vi "Start Kernel and Connect.vi"(6 "run minimized? (F)":bool=TRUE, 8 "error in (no error)":errorcluster, 9 "args":string="kernel   -f ", 10 "Path to Kernel Command (IPython)":string="\n", 11 "object in":refnum<class "JuPyter_Client.lvclass">) -> (0 "error out":errorcluster, 3 "object out":refnum<class "JuPyter_Client.lvclass">)   [LabVIEW 2018, in "JuPyter_Client.lvclass"]
doc: "Connect to an existing kernel"
uses:
  JuPyter_Client.lvclass
  Utility/Connection.ctl
  JuPyter_Client.lvclass/JuPyter_Client.ctl
  <vilib>/addons/zeromq/socket_type.ctl
  <vilib>/addons/zeromq/socket_options.ctl
  <vilib>/addons/zeromq/zmq_socket.lvclass
  <vilib>/addons/zeromq/zmq_context.lvclass
  <vilib>/addons/zeromq/zeromq.lvlib
  ClientMessaging.lvlib
  <vilib>/JDP Science/JSONtext/JSONtext.lvlib
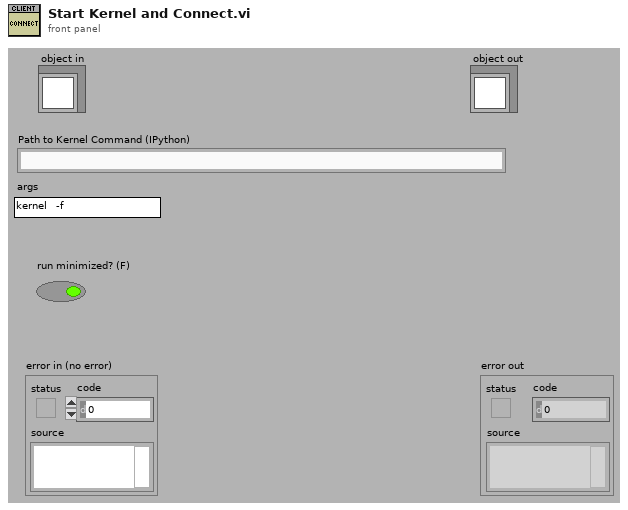
[diagram p1: front panel]
types:
  T1 = typedef "ClientMessaging.lvlib/Connection.ctl" = cluster{"transport":string, "ip":string, "key":string, "signature_scheme":string, "kernel_name":string, "shell_port":u16, "iopub_port":u16, "stdin_port":u16, "control_port":u16, "hb_port":u16}
  T2 = enum16{"Shell", "IOPub", "Stdin", "Control", "Heart Beat"}
  T3 = typedef "zeromq.lvlib/socket_type.ctl" = enum8{"ZMQ_PAIR", "ZMQ_PUB", "ZMQ_SUB", "ZMQ_REQ", "ZMQ_REP", "ZMQ_DEALER", "ZMQ_ROUTER", "ZMQ_PULL", "ZMQ_PUSH", "ZMQ_XPUB", "ZMQ_XSUB"}
  T4 = typedef "zeromq.lvlib/socket_options.ctl" = enum8{"NONE", "ZMQ_HWM", "<2>", "ZMQ_SWAP", "ZMQ_AFFINITY", "ZMQ_IDENTITY", "ZMQ_SUBSCRIBE", "ZMQ_UNSUBSCRIBE", "ZMQ_RATE", "ZMQ_RECOVERY_IVL", "ZMQ_MCAST_LOOP", "ZMQ_SNDBUF", "ZMQ_RCVBUF", "ZMQ_RCVMORE", "ZMQ_FD", "ZMQ_EVENTS", "ZMQ_TYPE", "ZMQ_LINGER", "ZMQ_RECONNECT_IVL", "ZMQ_BACKLOG", "ZMQ_RECOVERY_IVL_MSEC", "ZMQ_RECONNECT_IVL_MAX", "ZMQ_MAXMSGSIZE", "ZMQ_SNDHWM", "ZMQ_RCVHWM", "ZMQ_MULTICAST_HOPS", "<26>", "ZMQ_RCVTIMEO", "ZMQ_SNDTIMEO", "<29>", "<30>", "ZMQ_IPV4ONLY", "ZMQ_LAST_ENDPOINT", "ZMQ_ROUTER_MANDATORY", "ZMQ_TCP_KEEPALIVE", "ZMQ_TCP_KEEPALIVE_CNT", "ZMQ_TCP_KEEPALIVE_IDLE", "ZMQ_TCP_KEEPALIVE_INTVL", "ZMQ_TCP_ACCEPT_FILTER", "ZMQ_DELAY_ATTACH_ON_CONNECT", "ZMQ_XPUB_VERBOSE"}
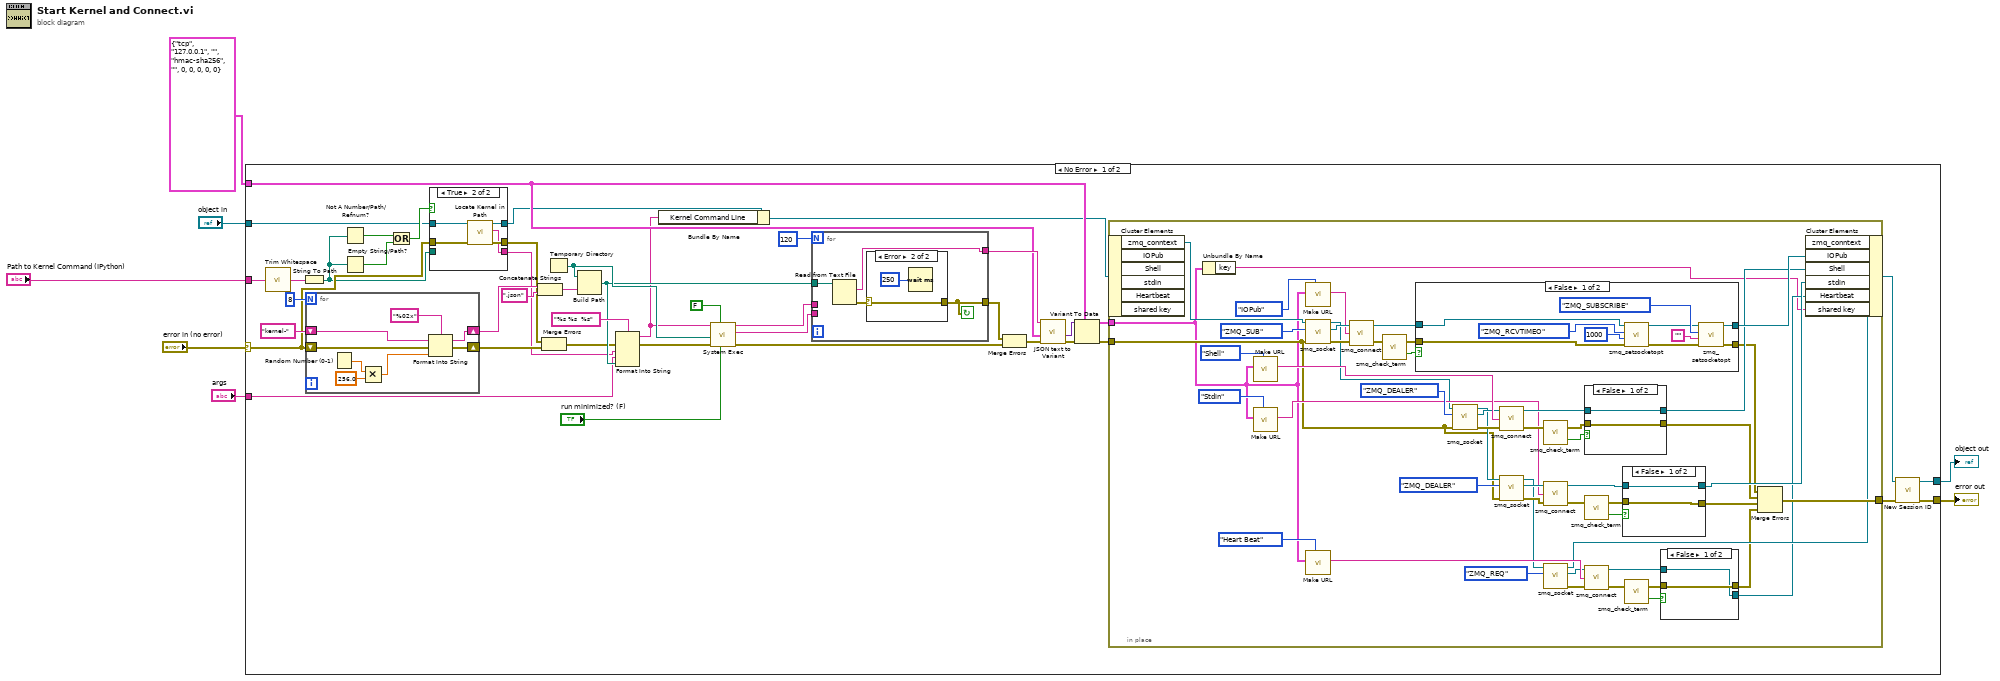
[diagram p0: block diagram]
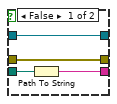
[diagram p2: hidden frame]
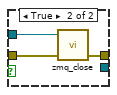
[diagram p4: hidden frame]
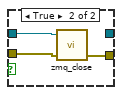
[diagram p5: hidden frame]
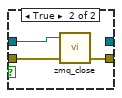
[diagram p6: hidden frame]
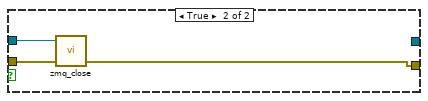
[diagram p7: hidden frame]
diagram:
  n1 = case shown="No Error" "error in (no error)" {
    selector: "error in (no error)" -> [w16 w157]
    tunnel: [w47 w157] -> w6
    tunnel: [w49 w156] -> w4
    tunnel: "object in" -> [w17 w156]
    tunnel: T1 {"transport"="tcp", "ip"="127.0.0.1", "key"="", "signature_scheme"="hmac-sha256", "kernel_name"="", "shell_port"=0, "iopub_port"=0, "stdin_port"=0, "control_port"=0, "hb_port"=0} ("Connection Info") -> [w32 _]
    tunnel: "Path to Kernel Command (IPython)" -> [w26 _]
    tunnel: "args" -> [w22 _]
    frame No Error {
      n2 = call <vilib>:"Trim Whitespace.vi"("string"=w26) -> ("trimmed string"=w8:string)  [unwired: 1 in]
      n3 = String To Path(string=w8) -> (path=w12:path)
      n4 = for {
        N: 8 -> [_]
        shift-right: [w72] -> w44
        shift-left: "kernel-" ("command line") -> [w71]
        shift-right: [w67] -> w37
        shift-left: w16 -> [w68]
        n5 = Random Number (0-1)() -> (number: 0 to 1=w74:dbl)
        n6 = Multiply(x=w74, y=256.0) -> (x*y=w70:dbl)
        n7 = Format Into String(format string="%02x", initial string=w71, error in=w68, w70) -> (resulting string=w72:string, error out=w67:errorcluster)
      }
      n8 = Not A Number/Path/Refnum?(number/path/refnum=w12) -> (NaN/Path/Refnum?=w21:bool)
      n9 = Empty String/Path?(string/path=w12) -> (empty?=w20:bool)
      n10 = Or(x=w21, y=w20) -> (x .or. y?=w19:bool)
      n11 = case shown="True" w19 {
        tunnel: w17 -> [w54 w59]
        tunnel: [w54 w58] -> w18
        tunnel: w16 -> [w53 w57]
        tunnel: [w53 w56] -> w14
        tunnel: [w51 w55] -> w13
        tunnel: w12 -> [w52 _]
        frame False {
          n12 = Path To String(path=w52) -> (string=w51:string)
        }
        frame True {
          n13 = call "Locate Kernel in Path.vi"("error in (no error)"=w57, "object in"=w59) -> ("error out"=w56:errorcluster, "Path to ipython"=w55:string, "object out"=w58:refnum<class "JuPyter_Client.lvclass">)  [unwired: 7 in]
        }
      }
      n14 = Concatenate Strings(w44, ".json") -> (w38:string)
      n15 = Merge Errors(w14, w37) -> (w15:errorcluster)
      n16 = Temporary Directory() -> (w39:path)
      n17 = Build Path(base path=w39, name or relative path=w38) -> (appended path=w23:path)
      n18 = Format Into String(format string="%s %s  %s", error in=w15, w13, w22, w23) -> (resulting string=w10:string, error out=w40:errorcluster)  [unwired: 1 in]
      n19 = Bundle By Name(cluster=w18, "Kernel Command Line"=w10) -> (w11:refnum<class "JuPyter_Client.lvclass">)
      n20 = call <vilib>:"System Exec.vi"("run minimized? (F)"="run minimized? (F)", "wait until completion? (T)"=FALSE, "error in (no error)"=w40, "working directory"=w39, "command line"=w10) -> ("error out"=w27:errorcluster, "standard error"=w24:string, "standard output"=w25:string)  [unwired: 3 in, 1 out]
      n21 = for {
        N: 120 -> [_]
        tunnel: w23 -> [w63]
        tunnel: [w61] -> w35
        tunnel: [w60] -> w29
        tunnel: w25 -> [_]
        tunnel: w24 -> [_]
        stop <- w60 continue-if-true
        n22 = Read from Text File(file (use dialog)=w63) -> (text=w61:string, error out=w62:errorcluster)  [unwired: 3 in, 2 out]
        n23 = case shown="Error" w62 {
          selector: w62 -> [w64 w66]
          tunnel: [w64 w66] -> w60
          frame No Error {
          }
          frame Error {
            n24 = Wait (ms)(milliseconds to wait=u32 250) -> ()  [unwired: 1 out]
          }
        }
      }
      n25 = Merge Errors(w29, w27) -> (w28:errorcluster)
      n26 = call <vilib>:"JSON text to Variant.vi"("error in (no error)"=w28, "Data Type"=w32, "JSON"=w35) -> ("error out"=w34:errorcluster, "Variant out"=w33:variant)  [unwired: 7 in]
      n27 = Variant To Data(error in=w34, type=w32, Variant=w33) -> (data=w31:T1, error out=w30:errorcluster)
      n28 = in-place {
        in-place-border: w31 -> [w76]
        in-place-border: w30 -> [w96]
        in-place-border: [w90] -> w48
        n29 = in-place-cluster #1(w11) -> ("zmq_conntext"=w127:refnum<class "zmq_context.lvclass">)  [unwired: 5 out]
        n30 = Unbundle By Name(w76) -> ("key"=w75:string)
        n31 = call "Make URL.vi"("Port"=T2."Shell", "Connection Info"=w76) -> ("Connection URL"=w112:string)  [unwired: 9 in]
        n32 = call "Make URL.vi"("Port"=T2."Stdin", "Connection Info"=w76) -> ("Connection URL"=w107:string)  [unwired: 9 in]
        n33 = call "Make URL.vi"("Port"=T2."IOPub", "Connection Info"=w76) -> ("Connection URL"=w124:string)  [unwired: 9 in]
        n34 = call <vilib>:"zmq_socket.vi"("error in"=w96, "socket type"=socket_type."ZMQ_SUB", "context in"=w127) -> ("error out"=w123:errorcluster, "socket out"=w125:refnum<class "zmq_socket.lvclass">, "context out"=w101:refnum<class "zmq_context.lvclass">)  [unwired: 2 in]
        n35 = call "Make URL.vi"("Port"=T2."Heart Beat", "Connection Info"=w76) -> ("Connection URL"=w83:string)  [unwired: 9 in]
        n36 = call <vilib>:"zmq_connect.vi"("error in"=w123, "endpoint"=w124, "socket in"=w125) -> ("error out"=w122:errorcluster, "socket out"=w120:refnum<class "zmq_socket.lvclass">)  [unwired: 1 in]
        n37 = call <vilib>:"zmq_check_term.vi"("error in"=w122) -> ("term?"=w121:bool, "error out"=w119:errorcluster)  [unwired: 1 in]
        n38 = case shown="False" w121 {
          tunnel: w120 -> [w147 w155]
          tunnel: w119 -> [w148 w154]
          tunnel: [w150 w153] -> w93
          tunnel: [w152 _] -> w118
          frame False {
            n39 = call <vilib>:"zmq_setsocketopt.vi"("error in"=w148, "value"=1000, "option"=socket_options."ZMQ_RCVTIMEO", "socket in"=w147) -> ("error out"=w146:errorcluster, "socket out"=w145:refnum<class "zmq_socket.lvclass">)  [unwired: 2 in]
            n40 = call <vilib>:"zmq_setsocketopt.vi"("error in"=w146, "value"="", "option"=socket_options."ZMQ_SUBSCRIBE", "socket in"=w145) -> ("error out"=w150:errorcluster, "socket out"=w152:refnum<class "zmq_socket.lvclass">)  [unwired: 2 in]
          }
          frame True {
            n41 = call <vilib>:"zmq_close.vi"("error in"=w154, "socket"=w155) -> ("error out"=w153:errorcluster)  [unwired: 3 in]
          }
        }
        n42 = call <vilib>:"zmq_socket.vi"("error in"=w96, "socket type"=socket_type."ZMQ_DEALER", "context in"=w101) -> ("error out"=w113:errorcluster, "socket out"=w111:refnum<class "zmq_socket.lvclass">, "context out"=w100:refnum<class "zmq_context.lvclass">)  [unwired: 2 in]
        n43 = call <vilib>:"zmq_connect.vi"("error in"=w113, "endpoint"=w112, "socket in"=w111) -> ("error out"=w114:errorcluster, "socket out"=w116:refnum<class "zmq_socket.lvclass">)  [unwired: 1 in]
        n44 = call <vilib>:"zmq_socket.vi"("error in"=w96, "socket type"=socket_type."ZMQ_DEALER", "context in"=w100) -> ("error out"=w106:errorcluster, "socket out"=w108:refnum<class "zmq_socket.lvclass">, "context out"=w80:refnum<class "zmq_context.lvclass">)  [unwired: 2 in]
        n45 = call <vilib>:"zmq_check_term.vi"("error in"=w114) -> ("term?"=w115:bool, "error out"=w117:errorcluster)  [unwired: 1 in]
        n46 = call <vilib>:"zmq_connect.vi"("error in"=w106, "endpoint"=w107, "socket in"=w108) -> ("error out"=w105:errorcluster, "socket out"=w103:refnum<class "zmq_socket.lvclass">)  [unwired: 1 in]
        n47 = call <vilib>:"zmq_socket.vi"("socket type"=socket_type."ZMQ_REQ", "context in"=w80) -> ("error out"=w84:errorcluster, "socket out"=w82:refnum<class "zmq_socket.lvclass">, "context out"=w79:refnum<class "zmq_context.lvclass">)  [unwired: 3 in]
        n48 = case shown="False" w115 {
          tunnel: w116 -> [w138 w142]
          tunnel: w117 -> [w139 w141]
          tunnel: [w139 w140] -> w92
          tunnel: [w138 _] -> w95
          frame False {
          }
          frame True {
            n49 = call <vilib>:"zmq_close.vi"("error in"=w141, "socket"=w142) -> ("error out"=w140:errorcluster)  [unwired: 3 in]
          }
        }
        n50 = call <vilib>:"zmq_check_term.vi"("error in"=w105) -> ("term?"=w104:bool, "error out"=w102:errorcluster)  [unwired: 1 in]
        n51 = call <vilib>:"zmq_connect.vi"("error in"=w84, "endpoint"=w83, "socket in"=w82) -> ("error out"=w85:errorcluster, "socket out"=w87:refnum<class "zmq_socket.lvclass">)  [unwired: 1 in]
        n52 = case shown="False" w104 {
          tunnel: w103 -> [w133 w137]
          tunnel: w102 -> [w134 w136]
          tunnel: [w134 w135] -> w91
          tunnel: [w133 _] -> w94
          frame False {
          }
          frame True {
            n53 = call <vilib>:"zmq_close.vi"("error in"=w136, "socket"=w137) -> ("error out"=w135:errorcluster)  [unwired: 3 in]
          }
        }
        n54 = call <vilib>:"zmq_check_term.vi"("error in"=w85) -> ("term?"=w86:bool, "error out"=w88:errorcluster)  [unwired: 1 in]
        n55 = case shown="False" w86 {
          tunnel: w87 -> [w128 w132]
          tunnel: w88 -> [w129 w131]
          tunnel: [w129 w130] -> w77
          tunnel: [w128 _] -> w78
          frame False {
          }
          frame True {
            n56 = call <vilib>:"zmq_close.vi"("error in"=w131, "socket"=w132) -> ("error out"=w130:errorcluster)  [unwired: 3 in]
          }
        }
        n57 = Merge Errors(w93, w92, w91, w77) -> (w90:errorcluster)
        n58 = in-place-cluster #1("zmq_conntext"=w79, "IOPub"=w118, "Shell"=w95, "stdin"=w94, "Heartbeat"=w78, "shared key"=w75) -> (w50:refnum<class "JuPyter_Client.lvclass">)
      }
      n59 = call-dynamic "New Session ID.vi"("error in (no error)"=w48, "object in"=w50) -> ("error out"=w47:errorcluster, "object out"=w49:refnum<class "JuPyter_Client.lvclass">)  [unwired: 8 in]
    }
    frame Error {
    }
  }
  "error out" <- w6
  "object out" <- w4
